vi "Servo Tester.vi"() -> ()   [LabVIEW 2020]
uses:
  <vilib>/DAQmx/create/channels.llb/DAQmx Create Channel (CO-Pulse Generation-Frequency).vi
  <vilib>/DAQmx/configure/timing.llb/DAQmx Timing (Implicit).vi
  <resource>/objmgr/daqmx.rc
panel:
  out "loop time (ms)":dbl
  in  "counter":tag
  in  "stop":bool
  in  "frequency":dbl=300.0 format="%#_13g"
  in  "pulse width (us)":dbl=5.0 format="%_6g"
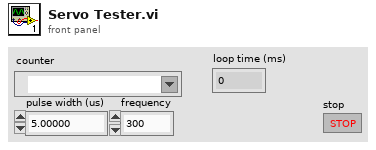
[diagram p1: front panel]
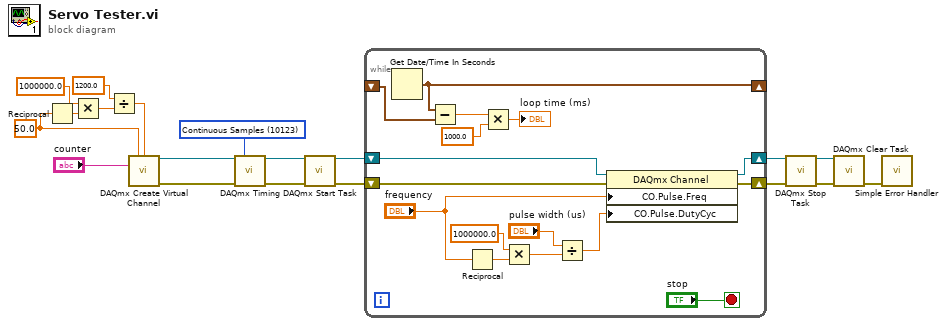
[diagram p0: block diagram]
diagram:
  w6 = 50.0 ("frequency")
  w12 = 10123 items=["Finite Samples"=10178, "Continuous Samples"=10123, "Hardware Timed Single Point"=12522] ("sample mode")
  n1 = Reciprocal(x=w6) -> (1/x=w5:dbl)
  n2 = Multiply(x=1000000.0, y=w5) -> (x*y=w3:dbl)
  n3 = Divide(x=1200.0 ("duty cycle"), y=w3) -> (x/y=w1:dbl)
  n4 = call-poly <vilib>:"DAQmx Create Virtual Channel.vi"("frequency"=w6, "duty cycle"=w1, "counter"="counter") -> ("task out"=w11:refnum<k21>, "error out"=w10:errorcluster)  [unwired: 11 in]
  n5 = call-poly <vilib>:"DAQmx Timing.vi"("task/channels in"=w11, "sample mode"=w12, "error in"=w10) -> ("task out"=w8:refnum<k21>, "error out"=w9:errorcluster)  [unwired: 11 in]
  n6 = call <vilib>:"DAQmx Start Task.vi"("task/channels in"=w8, "error in"=w9) -> ("task out"=w17:refnum<k21>, "error out"=w16:errorcluster)  [unwired: 12 in]
  n7 = while {
    shift-right: [w31] -> w14
    shift-left: w17 -> [w32]
    shift-right: [w33] -> w15
    shift-left: w16 -> [w34]
    shift-right: [w30] -> _
    shift-left: _ -> [w29]
    stop <- "stop" stop-if-true
    n8 = Get Date/Time In Seconds() -> (seconds since 1Jan1904=w30:timestamp)
    n9 = Subtract(x=w30, y=w29) -> (x-y=w28:dbl)
    n10 = Reciprocal(x="frequency") -> (1/x=w23:dbl)
    n11 = Multiply(x=w28, y=1000.0) -> (x*y=→"loop time (ms)":dbl)
    n12 = Multiply(x=1000000.0, y=w23) -> (x*y=w25:dbl)
    n13 = Divide(x="pulse width (us)", y=w25) -> (x/y=w20:dbl)
    n14 = property class="DAQmx Channel"(reference=w32, error in=w34, "CO.Pulse.Freq"="frequency", "CO.Pulse.DutyCyc"=w20) -> (reference out=w31:refnum<k21>, error out=w33:errorcluster)
  }
  n15 = call <vilib>:"DAQmx Stop Task.vi"("task/channels in"=w14, "error in"=w15) -> ("task out"=w18:refnum<k21>, "error out"=w19:errorcluster)  [unwired: 12 in]
  n16 = call <vilib>:"DAQmx Clear Task.vi"("task in"=w18, "error in"=w19) -> ("error out"=w7:errorcluster)  [unwired: 13 in]
  n17 = call <vilib>:"Simple Error Handler.vi"("error in (no error)"=w7) -> ()  [unwired: 4 in, 5 out]
